vi "Add 1Row.vi"(8 "error in (no error)":errorcluster, 10 "1 Row Names":string[](array[string]), 11 "MCLB_Lib in":refnum<class "MCLB_Lib.lvclass">) -> (0 "error out":errorcluster, 3 "MCLB_Lib out":refnum<class "MCLB_Lib.lvclass">)   [LabVIEW 2020, in "MCLB_Lib.lvclass"]
uses:
  MCLB_Lib.lvclass
  <vilib>/Utility/miscctls.llb/LVRowAndColumnUnsignedTypeDef.ctl
  MCLB_Lib.lvclass/MCLB_Lib.ctl
  7c460c6b-a38e-4a94-bb65-dd6f5ae24c8c.vi
  e68b9a2f-bd94-4d5c-86c4-a9e432a33499.vi
  <vilib>/Comparison/Equal/Equal Functor/Equal Functor.lvclass
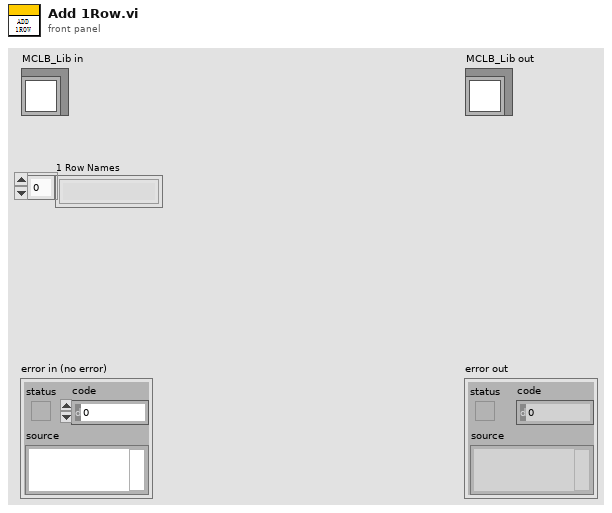
[diagram p1: front panel]
types:
  T1 = typedef "LVRowAndColumnUnsignedTypeDef.ctl" = cluster{"Row":u32, "Column":u32}
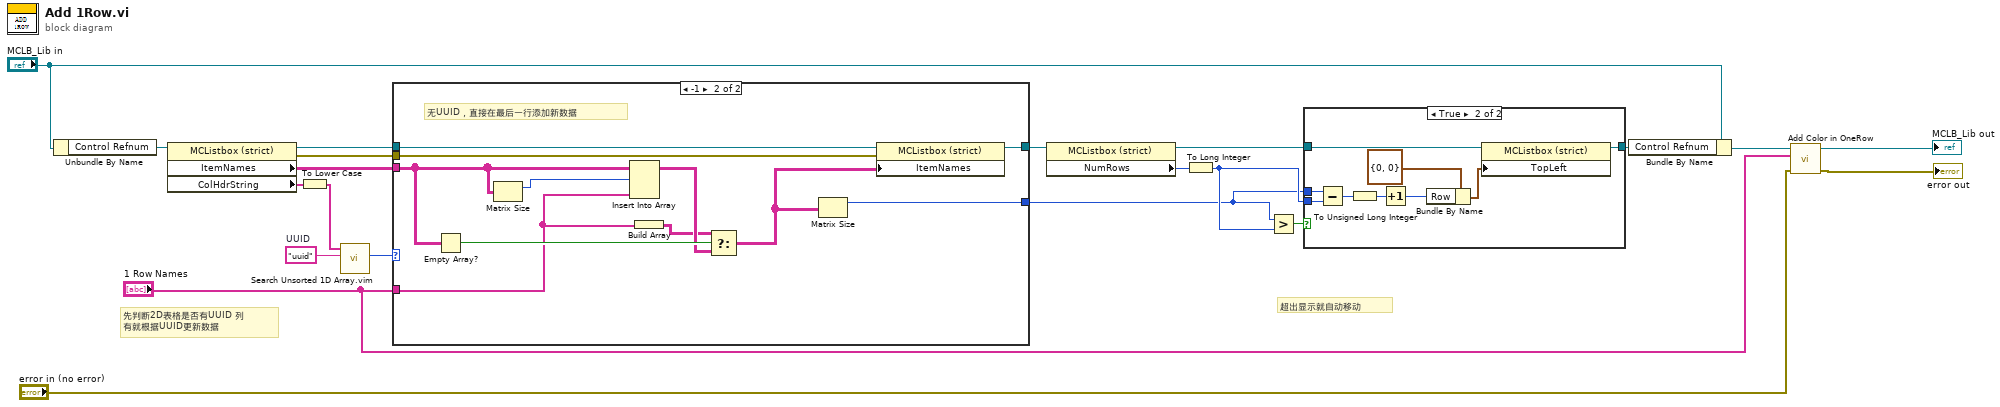
[diagram p0: block diagram]
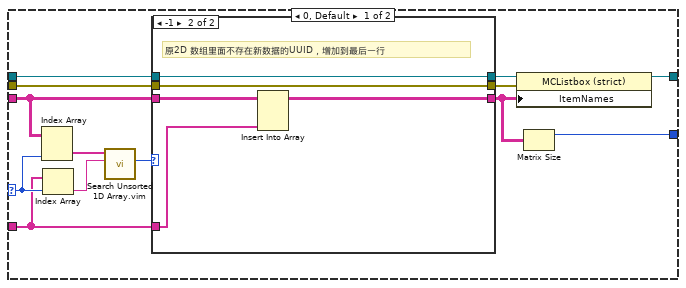
[diagram p3: hidden frame]
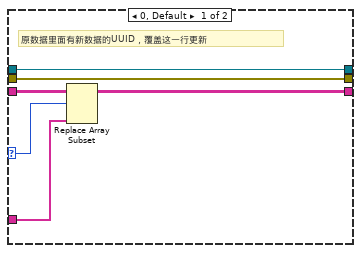
[diagram p4: hidden frame]
diagram:
  w19 = "uuid"  # UUID
  # "超出显示就自动移动"
  # "先判断2D表格是否有UUID 列\n有就根据UUID更新数据"
  n1 = Unbundle By Name("MCLB_Lib in") -> ("Control Refnum"=w20:refnum<vi>)
  n2 = property class="MCListbox (strict)"(reference=w20) -> (reference out=w16:refnum<vi>, error out=w15:errorcluster, "ItemNames"=w18:string[][], "ColHdrString"=w14:string[])  [unwired: 1 in]
  n3 = To Lower Case(string=w14) -> (all lower case string=w8:string[])
  n4 = call "Search Unsorted 1D Array.vim"("element"=w19, "unsorted 1D array"=w8) -> ("index of element"=w17:i32)  [unwired: 9 in]
  n5 = case shown="-1" w17 {
    selector: w17 -> [w34 _]
    tunnel: "1 Row Names" -> [w28 w47]
    tunnel: w18 -> [w29 w51]
    tunnel: [w27 w55] -> w2
    tunnel: w16 -> [w30 w56]
    tunnel: w15 -> [w24 w54]
    tunnel: [w22 w53] -> w3
    frame 0, Default {
      n6 = Index Array(array=w29, index (col)=w34) -> (element=w33:string[])  [unwired: 1 in]
      n7 = Index Array(array=w28, index=w34) -> (element=w32:string)
      n8 = call "Search Unsorted 1D Array.vim"("element"=w32, "unsorted 1D array"=w33) -> ("index of element"=w31:i32)  [unwired: 9 in]
      n9 = case shown="-1" w31 {
        selector: w31 -> [w38 _]
        tunnel: [w40 w45] -> w26
        tunnel: w30 -> [w40 w45]
        tunnel: w29 -> [w39 w44]
        tunnel: w28 -> [w37 w43]
        tunnel: [w36 w42] -> w23
        tunnel: [w35 w41] -> w25
        tunnel: w24 -> [w35 w41]
        frame 0, Default {
          # "原数据里面有新数据的UUID，覆盖这一行更新"
          n10 = Replace Array Subset(array=w39, new element=w37, index (row)=w38) -> (w36:string[][])  [unwired: 1 in]
        }
        frame -1 {
          # "原2D 数组里面不存在新数据的UUID，增加到最后一行"
          n11 = Insert Into Array(array=w44, new element=w43) -> (w42:string[][])  [unwired: 2 in]
        }
      }
      n12 = property class="MCListbox (strict)"(reference=w26, error in=w25, "ItemNames"=w23) -> (reference out=w27:refnum<vi>)  [unwired: 1 out]
      n13 = Matrix Size(0:w23) -> (1:w22:i32)  [unwired: 1 out]
    }
    frame -1 {
      # "无UUID，直接在最后一行添加新数据"
      n14 = Empty Array?(array=w51) -> (empty?=w50:bool)
      n15 = Matrix Size(0:w51) -> (1:w52:i32)  [unwired: 1 out]
      n16 = Insert Into Array(array=w51, index (row)=w52, new element=w47) -> (w49:string[][])  [unwired: 1 in]
      n17 = Build Array(w47) -> (w46:string[][])
      n18 = Select(t=w46, s=w50, f=w49) -> (s? t:f=w48:string[][])
      n19 = Matrix Size(0:w48) -> (1:w53:i32)  [unwired: 1 out]
      n20 = property class="MCListbox (strict)"(reference=w56, error in=w54, "ItemNames"=w48) -> (reference out=w55:refnum<vi>)  [unwired: 1 out]
    }
  }
  n21 = property class="MCListbox (strict)"(reference=w2) -> (reference out=w7:refnum<vi>, "NumRows"=w6:u32)  [unwired: 1 in, 1 out]
  n22 = To Long Integer(number=w6) -> (32bit integer=w4:i32)
  n23 = Greater?(x=w3, y=w4) -> (0:w5:bool)
  n24 = case shown="True" w5 {
    tunnel: w7 -> [w57 w66]
    tunnel: [w57 w65] -> w1
    tunnel: w3 -> [_ w62]
    tunnel: w4 -> [_ w61]
    frame False {
    }
    frame True {
      n25 = Subtract(x=w62, y=w61) -> (x-y=w60:i32)
      n26 = To Unsigned Long Integer(number=w60) -> (unsigned 32bit integer=w59:u32)
      n27 = Increment(x=w59) -> (x+1=w58:u32)
      n28 = Bundle By Name(cluster=T1 {"Row"=0, "Column"=0} ("Top Left Visible Cell"), "Row"=w58) -> (w63:T1)
      n29 = property class="MCListbox (strict)"(reference=w66, "TopLeft"=w63) -> (reference out=w65:refnum<vi>)  [unwired: 1 in, 1 out]
    }
  }
  n30 = Bundle By Name(cluster="MCLB_Lib in", "Control Refnum"=w1) -> (w13:refnum<class "MCLB_Lib.lvclass">)
  n31 = call "Add Color in OneRow.vi"("error in (no error)"="error in (no error)", "1 Row Data"="1 Row Names", "MCLB_Lib in"=w13) -> ("error out"=→"error out":errorcluster, "MCLB_Lib out"=→"MCLB_Lib out":refnum<class "MCLB_Lib.lvclass">)  [unwired: 7 in]
